vi "OP20_HOSE_TEST_11_27_59_AM.vi"() -> ()   [LabVIEW 2020]
panel:
  in  "OP20_HOSE_TEST":T1
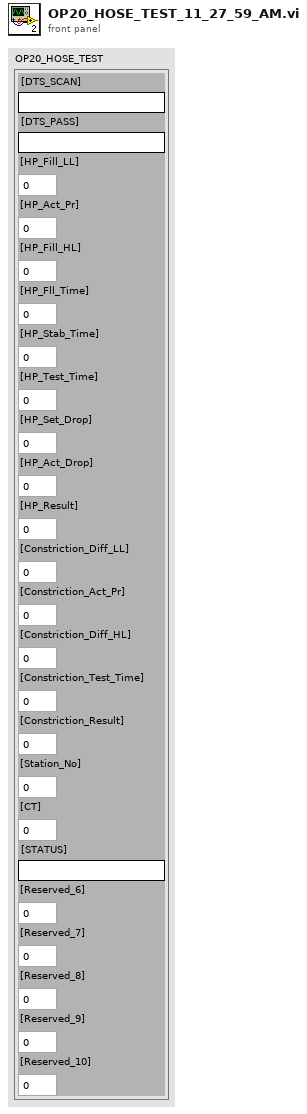
[diagram p1: front panel]
types:
  T1 = cluster{"[DTS_SCAN]":string, "[DTS_PASS]":string, "[HP_Fill_LL]":dbl, "[HP_Act_Pr]":dbl, "[HP_Fill_HL]":dbl, "[HP_Fll_Time]":dbl, "[HP_Stab_Time]":dbl, "[HP_Test_Time]":dbl, "[HP_Set_Drop]":dbl, "[HP_Act_Drop]":dbl, "[HP_Result]":dbl, "[Constriction_Diff_LL]":dbl, "[Constriction_Act_Pr]":dbl, "[Constriction_Diff_HL]":dbl, "[Constriction_Test_Time]":dbl, "[Constriction_Result]":dbl, "[Station_No]":dbl, "[CT]":dbl, "[STATUS]":string, "[Reserved_6]":dbl, "[Reserved_7]":dbl, "[Reserved_8]":dbl, "[Reserved_9]":dbl, "[Reserved_10]":dbl}
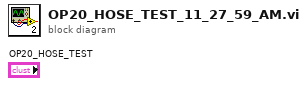
[diagram p0: block diagram]
diagram:
